vi "Get Use Alias.vi"(8 "error in (no error)":errorcluster, 11 "Node in":refnum<class "Node.lvclass">) -> (0 "error out":errorcluster, 2 "Use Alias":bool, 3 "Node out":refnum<class "Node.lvclass">)   [LabVIEW 2020, in "VolatusConfig.lvlib" / "Node.lvclass"]
uses:
  Node.lvclass
  Node.lvclass/Node.ctl
  VolatusConfigElement/VolatusConfigElement.lvclass
  lv-cdm/CDM-Config/Config Element/Config Element.lvclass
  C:/dev/lv20CE/relink/lv-volatus/VolatusConfig/VolatusConfigElement/VolatusConfigElement.lvclass
  C:/dev/lv20CE/relink/lv-volatus/VolatusConfig/Node/Node.lvclass
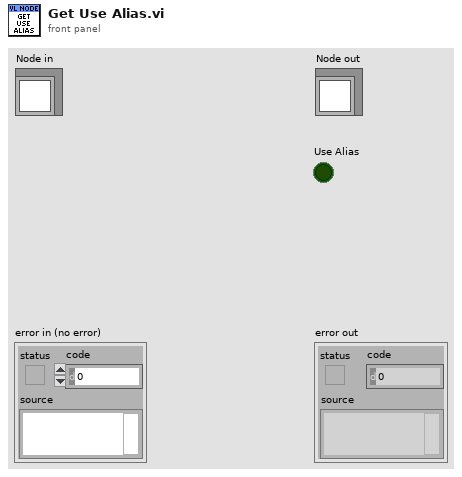
[diagram p1: front panel]
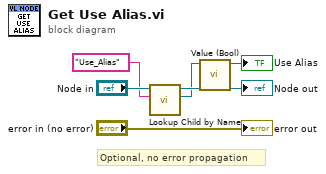
[diagram p0: block diagram]
diagram:
  # "Optional, no error propagation"
  n1 = call "Lookup Child by Name.vi"("Child Name"="Use_Alias", "VolatusConfigElement in"="Node in") -> ("Child"=w2:refnum<class "Config Element.lvclass">, "VolatusConfigElement out"=→"Node out":refnum<class "Node.lvclass">)  [unwired: 6 in, 2 out]
  n2 = call "Value (Bool).vi"("Config Element in"=w2) -> ("Bool Value"=→"Use Alias":bool)  [unwired: 9 in, 1 out]
  "error out" <- "error in (no error)"
